vi "NI-FGEN Specific Logic.vi"(7 "measurement configuration":T2={"pin_name"="", "waveform"=enum."Sine", "frequency"=6.0, "amplitude"=6.0, "duration"=6.0}, 8 "error in":errorcluster, 9 "channel list":string, 10 "session":refnum<k15>, 11 "measurement context":refnum<class "MeasurementContext.lvclass">) -> (0 "error out":errorcluster, 1 "measurement results":T1={"actual_duration"=1.0}, 2 "session out":refnum<k15>, 3 "measurement context out":refnum<class "MeasurementContext.lvclass">)   [LabVIEW 2020, in "NIFgenStandardFunction.lvlib"]
uses:
  NIFgenStandardFunction.lvlib
  Measurement Configuration.ctl
  Waveform.ctl
  Measurement Results.ctl
  <vilib>/MeasurementLink/MeasurementLink Measurement Server/Classes/MeasurementContext/MeasurementContext.lvclass
  <vilib>/MeasurementLink/MeasurementLink Measurement Server/Classes/MeasurementContext/Accessor/Is Canceled.vi
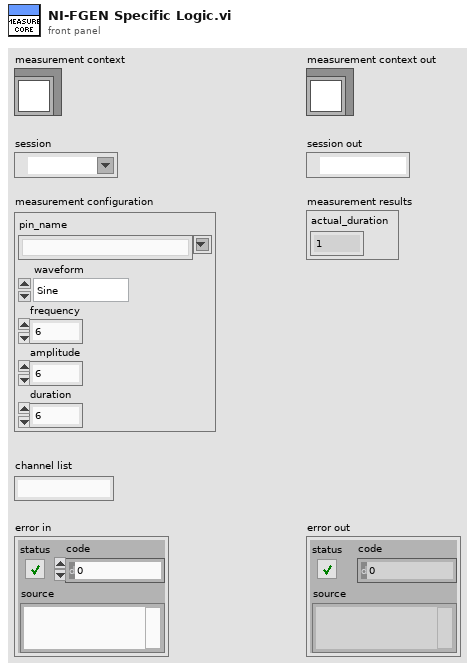
[diagram p1: front panel]
types:
  T1 = typedef "NIFgenStandardFunction.lvlib/Measurement Results.ctl" = cluster{"actual_duration":dbl}
  T2 = typedef "NIFgenStandardFunction.lvlib/Measurement Configuration.ctl" = cluster{"pin_name":string, "waveform":T3, "frequency":dbl, "amplitude":dbl, "duration":dbl}
  T3 = typedef "NIFgenStandardFunction.lvlib/Waveform.ctl" = enum16{"Sine", "Square", "Triangle", "Ramp Up", "Ramp Down", "DC", "Noise", "User"}
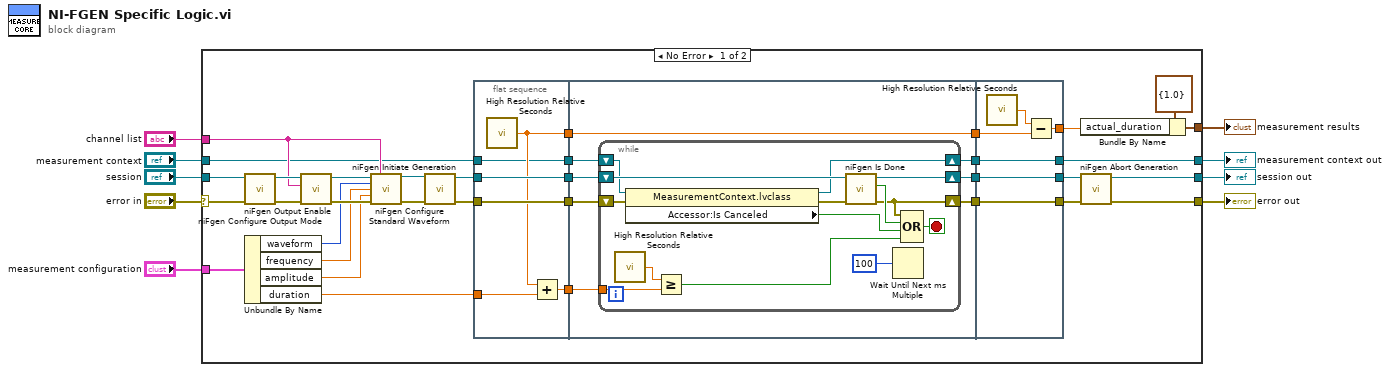
[diagram p0: block diagram]
diagram:
  n1 = case shown="No Error" "error in" {
    selector: "error in" -> [w43 w80]
    tunnel: "measurement configuration" -> [w41 _]
    tunnel: "session" -> [w42 w79]
    tunnel: "channel list" -> [w33 _]
    tunnel: [w25 w80] -> w5
    tunnel: [w24 w79] -> w4
    tunnel: [w22 _] -> w3
    tunnel: "measurement context" -> [w13 w78]
    tunnel: [w11 w78] -> w1
    frame No Error {
      n2 = call <instrlib>:"niFgen Configure Output Mode.vi"("error in (no error)"=w43, "Instrument Handle"=w42) -> ("error out"=w39:errorcluster, "Instrument Handle Out"=w40:refnum<k15>)  [unwired: 7 in]
      n3 = Unbundle By Name(w41) -> ("waveform"=w36:T3, "frequency"=w35:dbl, "amplitude"=w34:dbl, "duration"=w28:dbl)
      n4 = call <instrlib>:"niFgen Output Enable.vi"("error in (no error)"=w39, "Channel Name"=w33, "Instrument Handle"=w40) -> ("error out"=w38:errorcluster, "Instrument Handle Out"=w37:refnum<k15>)  [unwired: 7 in]
      n5 = call <instrlib>:"niFgen Configure Standard Waveform.vi"("Instrument Handle"=w37, "Channel Name"=w33, "Waveform"=w36, "Frequency"=w35, "Amplitude"=w34, "error in (no error)"=w38) -> ("Instrument Handle Out"=w32:refnum<k15>, "error out"=w31:errorcluster)  [unwired: 8 in]
      n6 = call <instrlib>:"niFgen Initiate Generation.vi"("error in (no error)"=w31, "Instrument Handle"=w32) -> ("error out"=w30:errorcluster, "Instrument Handle Out"=w29:refnum<k15>)  [unwired: 8 in]
      n7 = flat-sequence {
        tunnel: w28 -> [w47]
        tunnel: w29 -> [w48]
        tunnel: w30 -> [w49]
        tunnel: [w49] -> w21
        tunnel: [w48] -> w20
        tunnel: [w46] -> w19
        tunnel: [w45] -> w15
        tunnel: [w44] -> w14
        tunnel: w13 -> [w44]
        tunnel: w21 -> [w55]
        tunnel: w20 -> [w56]
        tunnel: w19 -> [w57]
        tunnel: [w54] -> w18
        tunnel: [w53] -> w17
        tunnel: [w57] -> w16
        tunnel: w15 -> [w52]
        tunnel: w14 -> [w51]
        tunnel: [w50] -> w12
        tunnel: [w76] -> w26
        tunnel: [w77] -> w27
        tunnel: w18 -> [w77]
        tunnel: w17 -> [w76]
        tunnel: w16 -> [w75]
        tunnel: [w74] -> w10
        tunnel: [w72] -> w11
        tunnel: w12 -> [w72]
        frame #0 {
          n8 = call <vilib>:"High Resolution Relative Seconds.vi"() -> ("relative seconds"=w46:dbl)
          n9 = Add(x=w46, y=w47) -> (x+y=w45:dbl)
        }
        frame #1 {
          n10 = while {
            shift-right: [w67] -> w53
            shift-left: w56 -> [w68]
            shift-right: [w60] -> w54
            shift-left: w55 -> [w62]
            tunnel: w52 -> [w71]
            shift-right: [w63] -> w50
            shift-left: w51 -> [w64]
            stop <- w65 stop-if-true
            n11 = call <vilib>:"High Resolution Relative Seconds.vi"() -> ("relative seconds"=w70:dbl)
            n12 = property class="MeasurementContext.lvclass"(reference=w64, error in=w62) -> (reference out=w63:refnum<class "MeasurementContext.lvclass">, error out=w61:errorcluster, "Accessor:Is Canceled"=w59:bool)
            n13 = Greater Or Equal?(x=w70, y=w71) -> (x >= y?=w58:bool)
            n14 = call <instrlib>:"niFgen Is Done.vi"("error in (no error)"=w61, "Instrument Handle"=w68) -> ("error out"=w60:errorcluster, "Done"=w66:bool, "Instrument Handle Out"=w67:refnum<k15>)  [unwired: 7 in]
            n15 = Wait Until Next ms Multiple(millisecond multiple=u32 100) -> ()  [unwired: 1 out]
            n16 = Compound Arithmetic op=OR(w60, w66, w59, w58) -> (w65:bool)
          }
        }
        frame #2 {
          n17 = call <vilib>:"High Resolution Relative Seconds.vi"() -> ("relative seconds"=w73:dbl)
          n18 = Subtract(x=w73, y=w75) -> (x-y=w74:dbl)
        }
      }
      n19 = Bundle By Name(cluster=T1 {"actual_duration"=1.0} ("measurement results"), "actual_duration"=w10) -> (w22:T1)
      n20 = call <instrlib>:"niFgen Abort Generation.vi"("error in (no error)"=w27, "Instrument Handle"=w26) -> ("error out"=w25:errorcluster, "Instrument Handle Out"=w24:refnum<k15>)  [unwired: 8 in]
    }
    frame Error {
    }
  }
  "error out" <- w5
  "session out" <- w4
  "measurement results" <- w3
  "measurement context out" <- w1
